vi "SW-mini.vi"(8 "error in (no error)":errorcluster, 10 "Integration Time (ms)":i32=1000 caption="Inter scan delay ms", 11 "Spectral Channel":i32) -> (0 "error out":errorcluster, 1 "Spectrum":T1, 2 "Spectrometer wavelengths":sgl[](array[numeric]), 3 "Readings":sgl[](array[numeric]))   [LabVIEW 2012]
uses:
  SpectrometerSpectraWiz.llb/StellarNet Globals.vi
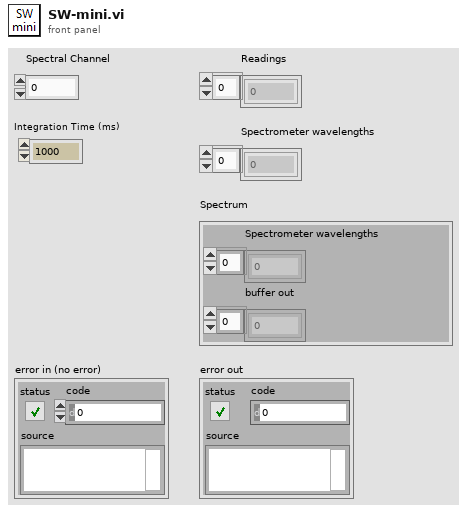
[diagram p1: front panel]
types:
  T1 = cluster{"Spectrometer wavelengths":sgl[], "buffer out":sgl[]}
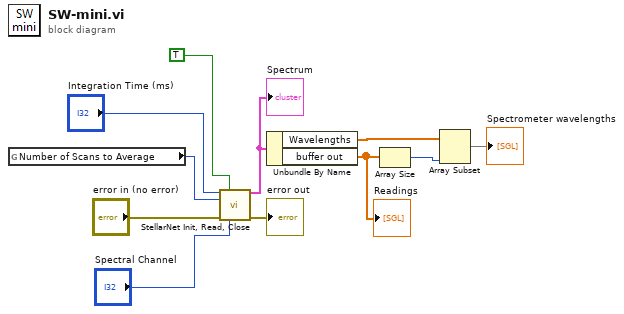
[diagram p0: block diagram]
diagram:
  n1 = global read "StellarNet Globals.vi" "Number of Scans to Average"() -> (w10:i32)
  n2 = call "StellarNet Init, Read, Close.vi"("Integration Time (ms)"="Integration Time (ms)", "Use Config\nFile Params (T)"=TRUE ("Use Config\nFile Params (T)"), "Number of Scans to Average"=w10, "error in (no error)"="error in (no error)", "Spectral Channel"="Spectral Channel") -> ("Spectrum"=w11:cluster{"Wavelengths":dbl[], "buffer out":sgl[]}, "error out"=→"error out":errorcluster)  [unwired: 7 in, 2 out]
  "Spectrum" <- w11
  n3 = Unbundle By Name(w11) -> ("Wavelengths"=w4:dbl[], "buffer out"=w3:sgl[])
  "Readings" <- w3
  n4 = Array Size(array=w3) -> (size(s)=w2:i32)
  n5 = Array Subset(array=w4, length=w2) -> (→"Spectrometer wavelengths":dbl[])  [unwired: 1 in]
